vi "SetDefaultAccelM1.vi"() -> ()   [LabVIEW 2015]
uses:
  <instrlib>/Ion Motion Roboclaw/Ion Motion Roboclaw.lvlib
panel:
  in  "Address":u8
  in  "Deccel":u32
  out "Valid":bool
  in  "Accel":u32
  out "error out":errorcluster
  in  "COM port":refnum<visa-resource-name>
  in  "baud rate (38400)":u32
  in  "error in (no error)":errorcluster
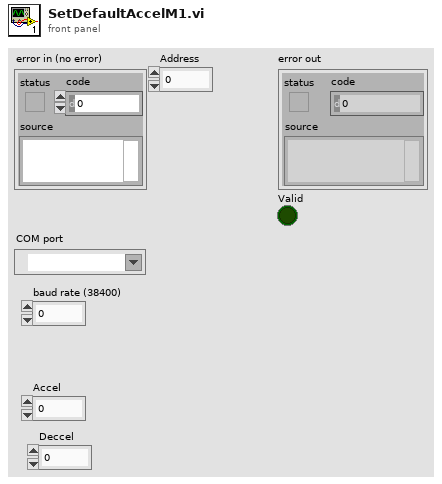
[diagram p1: front panel]
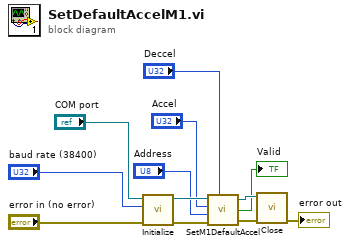
[diagram p0: block diagram]
diagram:
  n1 = call <instrlib>:"Initialize.vi"("error in (no error)"="error in (no error)", "baud rate (38400)"="baud rate (38400)", "COM port"="COM port") -> ("error out"=w11:errorcluster, "VISA resource name out"=w12:refnum<visa-resource-name>)  [unwired: 7 in]
  n2 = call <instrlib>:"SetM1DefaultAccel.vi"("VISA Refnum in"=w12, "Accel"="Accel", "Address"="Address", "error in (no error)"=w11, "Deccel"="Deccel") -> ("VISA Refnum out"=w10:refnum<visa-resource-name>, "Valid"=→"Valid":bool, "error out"=w9:errorcluster)
  n3 = call <instrlib>:"Close.vi"("error in (no error)"=w9, "VISA resource name"=w10) -> ("error out"=→"error out":errorcluster)  [unwired: 9 in]
